vi "MS SQL_InRFID_STN30C.vi"(6 "RFID":string, 7 "OP30C_007_SEAL_CHECK":T1, 8 "error in (no error)":errorcluster, 11 "Ref in":T2={"MS SQL Connection"=refnum, "UDL File"=path "", "Time"="", "DCODE"="", "WIP+1"=0, "MC No?"=0, "POKAYOKE?"=FALSE, "Expected Result"="", "Result [Status]"="", "Clock"=0.0, "RFID"="", "WIP Queue"=refnum, "TS Parameter"={"ProfitCenterCode"="", "LineCode"="", "WorkOrderNumber"="", "Model"="", "Model_with_Prefix"="", "VendorCode"="", "SetParameterDateCode"="", "PokaYoke"=0, "Target"=1, "Live_DateCode"="", "CustomerPartNumber"="", "Hand"="", "Ent_Stamp"=timestamp(0 s since 1904-01-01), "STS_CD"=0.0}, "Data_Queue"=[], "RFID Serial No."=""} {"TS Parameter"."Target" min=1 max=100000; "TS Parameter"."PokaYoke" min=0 max=1}) -> (0 "error out":errorcluster, 1 "Message":picture, 3 "Ref Out":T2={"MS SQL Connection"=refnum, "UDL File"=path "", "Time"="", "DCODE"="", "WIP+1"=0, "MC No?"=0, "POKAYOKE?"=FALSE, "Expected Result"="", "Result [Status]"="", "Clock"=0.0, "RFID"="", "WIP Queue"=refnum, "TS Parameter"={"ProfitCenterCode"="", "LineCode"="", "WorkOrderNumber"="", "Model"="", "Model_with_Prefix"="", "VendorCode"="", "SetParameterDateCode"="", "PokaYoke"=0, "Target"=1, "Live_DateCode"="", "CustomerPartNumber"="", "Hand"="", "Ent_Stamp"=timestamp(0 s since 1904-01-01), "STS_CD"=0.0}, "Data_Queue"=[], "RFID Serial No."=""} {"TS Parameter"."Target" min=1 max=100000; "TS Parameter"."PokaYoke" min=0 max=1})   [LabVIEW 2020]
uses:
  Controls/TD SQL.ctl
  <vilib>/addons/database/Connection.llb/Conn ObjectReference.ctl
  Controls/WIP_State.ctl
  Controls/TS_Parameter.ctl
  Controls/OP30C_DataCluster.ctl
  <vilib>/addons/database/NI_Database_API.lvlib
panel:
  out "resulting string":string
  # "OP60"
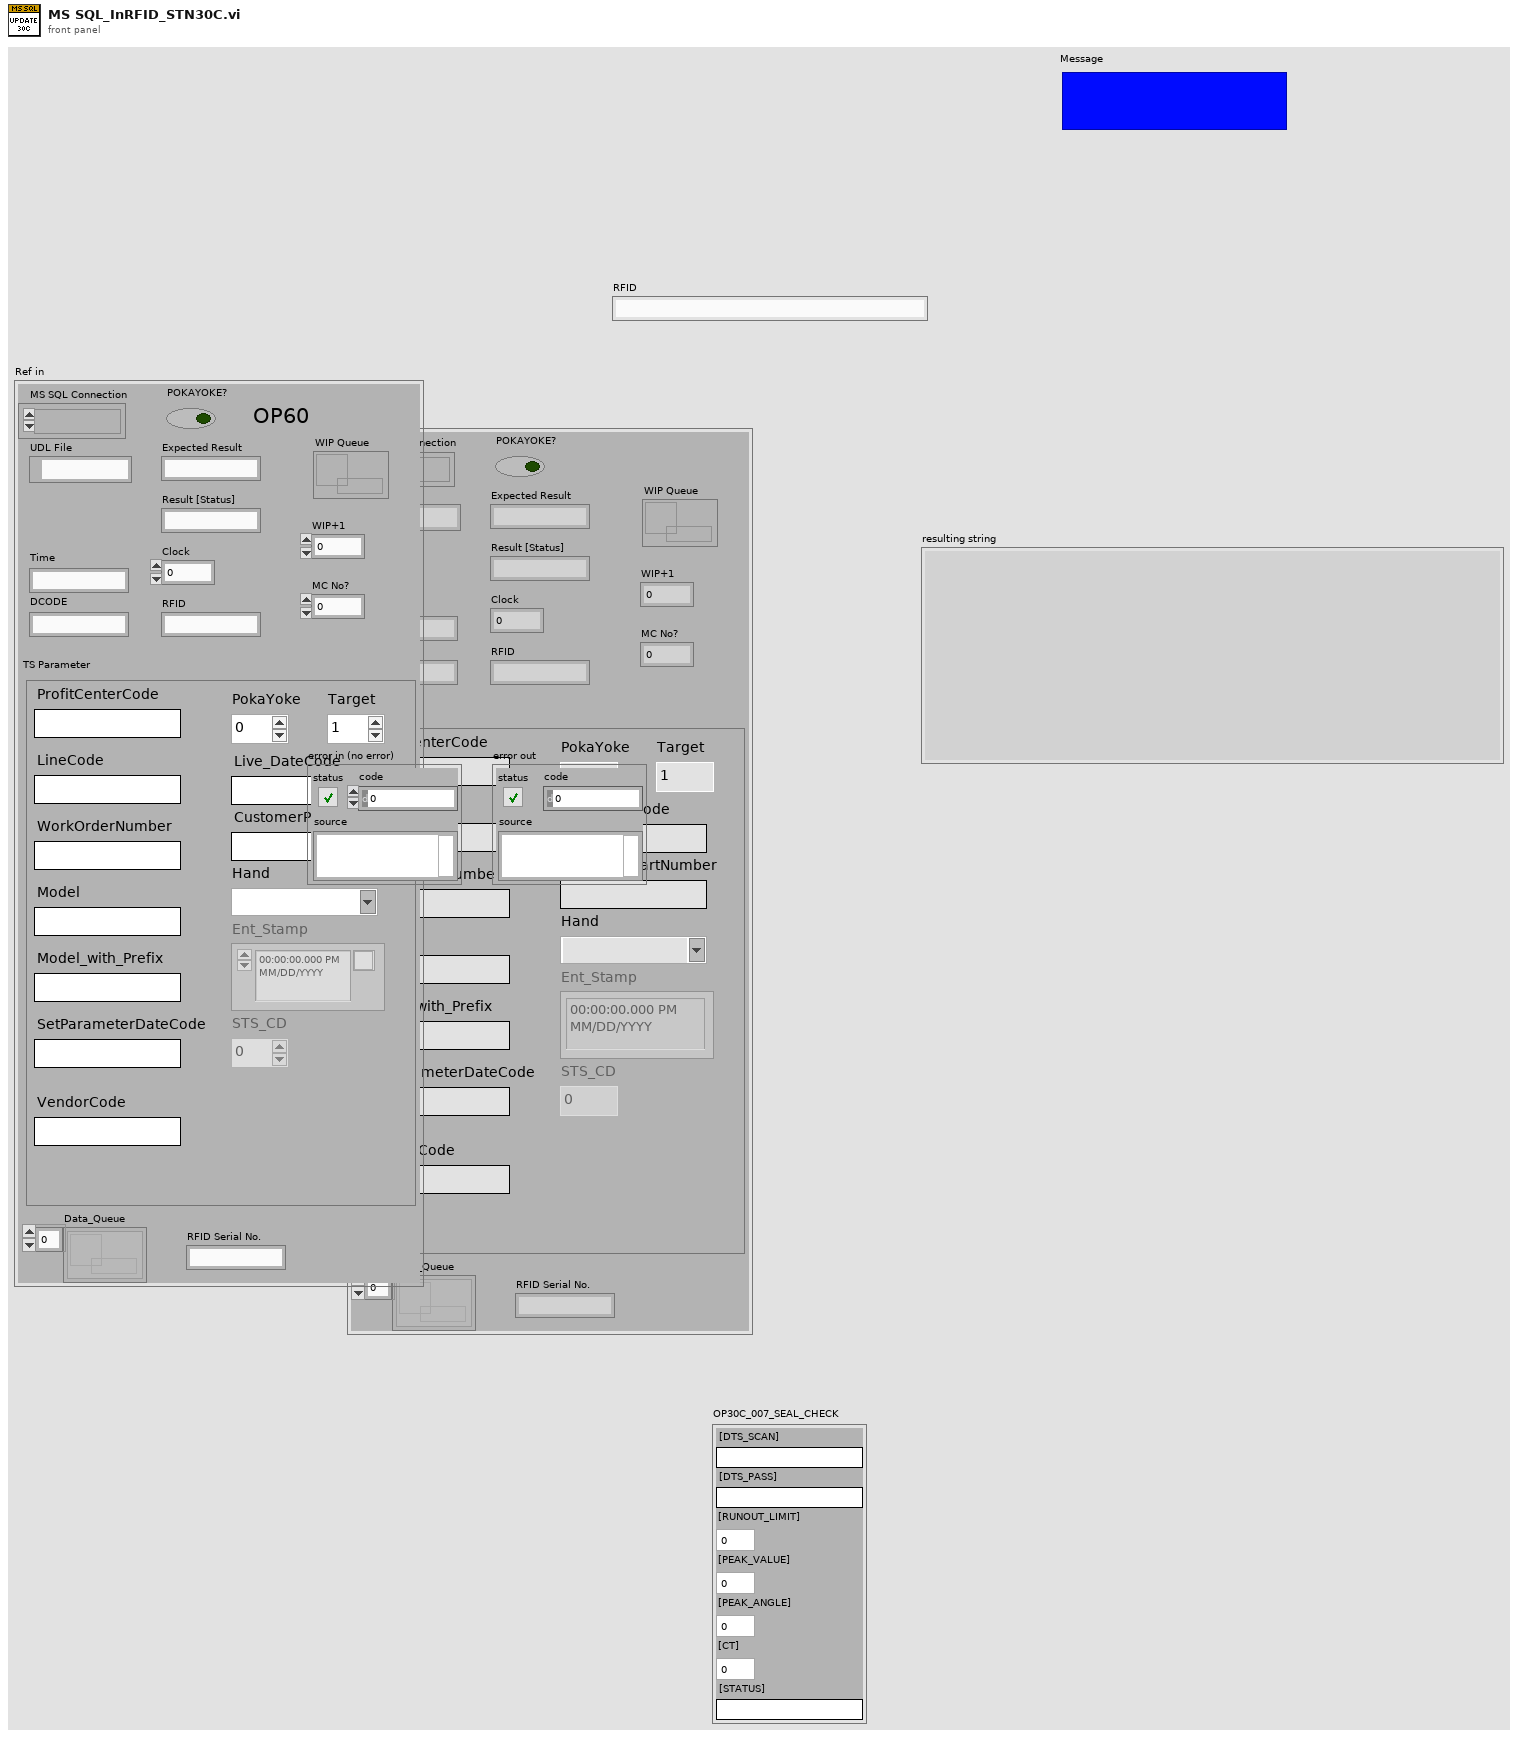
[diagram p1: front panel]
types:
  T1 = typedef "OP30C_DataCluster.ctl" = cluster{"[DTS_SCAN]":string, "[DTS_PASS]":string, "[RUNOUT_LIMIT]":dbl, "[PEAK_VALUE]":dbl, "[PEAK_ANGLE]":dbl, "[CT]":dbl, "[STATUS]":string}
  T2 = typedef "TD SQL.ctl" = cluster{"MS SQL Connection":T3, "UDL File":path, "Time":string, "DCODE":string, "WIP+1":i64, "MC No?":i32, "POKAYOKE?":bool, "Expected Result":string, "Result [Status]":string, "Clock":dbl, "RFID":string, "WIP Queue":refnum<queue>, "TS Parameter":T4, "Data_Queue":refnum<queue>[], "RFID Serial No.":string}
  T3 = typedef "NI_Database_API.lvlib/Conn ObjectReference.ctl" = refnum<k1>
  T4 = typedef "TS_Parameter.ctl" = cluster{"ProfitCenterCode":string, "LineCode":string, "WorkOrderNumber":string, "Model":string, "Model_with_Prefix":string, "VendorCode":string, "SetParameterDateCode":string, "PokaYoke":i32, "Target":i32, "Live_DateCode":string, "CustomerPartNumber":string, "Hand":string, "Ent_Stamp":timestamp, "STS_CD":dbl}
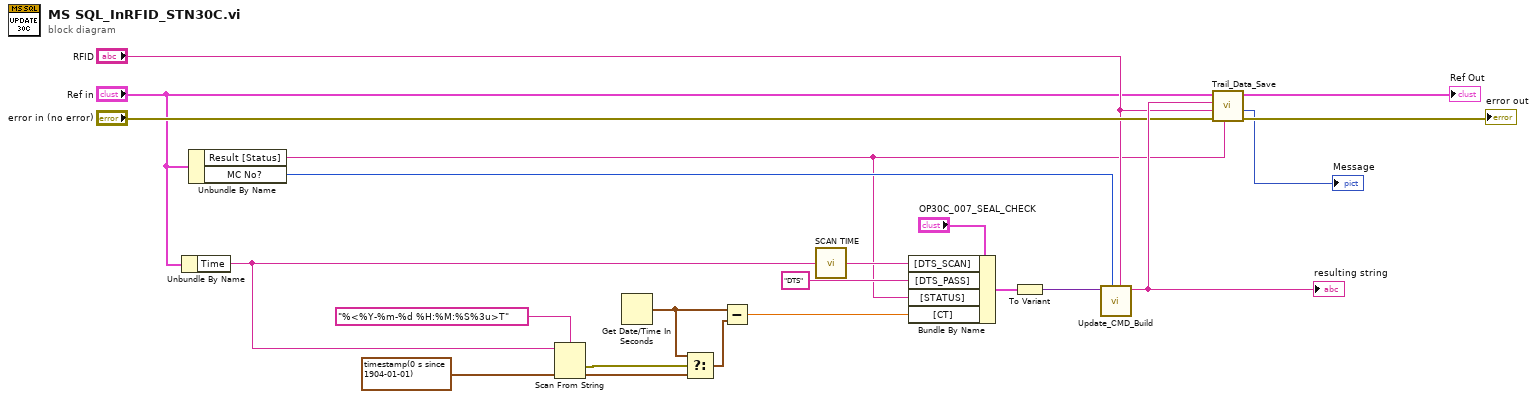
[diagram p0: block diagram]
diagram:
  n1 = Unbundle By Name("Ref in") -> ("Time"=w9:string)
  n2 = Unbundle By Name("Ref in") -> ("Result [Status]"=w1:string, "MC No?"=w2:i32)
  n3 = Scan From String(format string="%<%Y-%m-%d %H:%M:%S%3u>T", input string=w9, default 1=timestamp(0 s since 1904-01-01) ("Date Out")) -> (error out=w8:errorcluster, output 1=w6:timestamp)  [unwired: 2 in, 2 out]
  n4 = Get Date/Time In Seconds() -> (seconds since 1Jan1904=w7:timestamp)
  n5 = Select(t=w7, s=w8, f=w6) -> (s? t:f=w5:timestamp)
  n6 = Subtract(x=w7, y=w5) -> (x-y=w4:dbl)
  n7 = call "SCAN TIME.vi"("Time in"=w9) -> ("Time out"=w19:string)
  n8 = Bundle By Name(cluster="OP30C_007_SEAL_CHECK", "[DTS_SCAN]"=w19, "[DTS_PASS]"="DTS", "[STATUS]"=w1, "[CT]"=w4) -> (w22:T1)
  n9 = To Variant(anything=w22) -> (Variant=w20:variant)
  n10 = call "Update_CMD_Build.vi"("RFID"="RFID", "Machine No"=w2, "Variant"=w20) -> ("Update Query"=w17:string)  [unwired: 5 in, 1 out]
  "resulting string" <- w17
  n11 = call "Trail_Data_Save.vi"("Status"=w1, "error in (no error)"="error in (no error)", "RFID"="RFID", "Query"=w17, "Ref in"="Ref in") -> ("error out"=→"error out":errorcluster, "Message"=→"Message":picture, "Ref Out"=→"Ref Out":T2)  [unwired: 1 in, 1 out]
